vi "实验2_2（另一VI）.vi"() -> ()   [LabVIEW 2018]
panel:
  in  "delay":dbl format="%#_6f"
  out "ouput":dbl(graph)
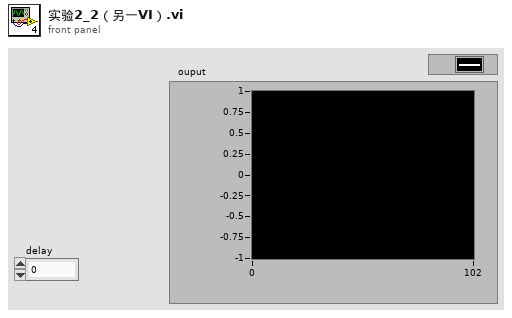
[diagram p1: front panel]
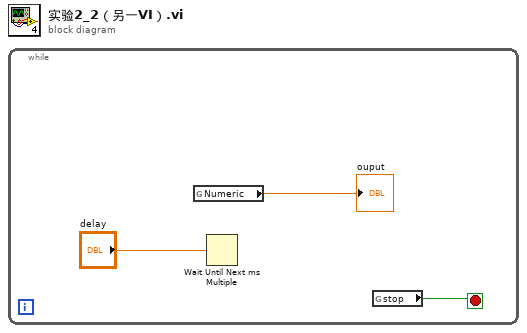
[diagram p0: block diagram]
diagram:
  n1 = while {
    stop <- w1 stop-if-true
    n2 = global read "实验2_2全局.vi" "Numeric"() -> (→"ouput":dbl)
    n3 = Wait Until Next ms Multiple(millisecond multiple="delay") -> ()  [unwired: 1 out]
    n4 = global read "实验2_2全局.vi" "stop"() -> (w1:bool)
  }
